vi "sort circles.vi"(1 "circles":T1(array[cluster])) -> (0 "Sorted circles":T1(array[cluster]))   [LabVIEW 2010]
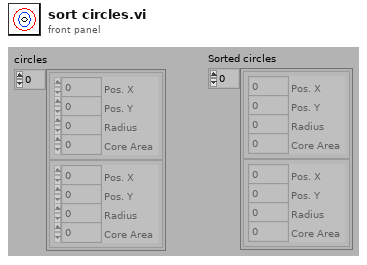
[diagram p1: front panel]
types:
  T1 = cluster{"Pos. X":i32, "Pos. Y":i32, "Radius":i32, "Core Area":i32}[]
  T2 = cluster{"Radius":i32, "Circles Data":cluster{"Pos. X":i32, "Pos. Y":i32, "Radius":i32, "Core Area":i32}}
  T3 = cluster{"Radius":i32, "Circles Data":cluster{"Pos. X":i32, "Pos. Y":i32, "Radius":i32, "Core Area":i32}}[]
  T4 = cluster{"Pos. X":i32, "Pos. Y":i32, "Radius":i32, "Core Area":i32}
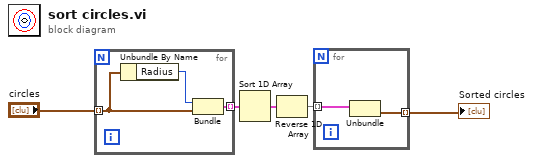
[diagram p0: block diagram]
diagram:
  n1 = for {
    tunnel: "circles" -> [w8] mode=indexing
    tunnel: [w7] -> w5 mode=indexing
    n2 = Unbundle By Name(w8) -> ("Radius"=w6:i32)
    n3 = Bundle("Radius"=w6, "Circles Data"=w8) -> (w7:T2)  [unwired: 1 in]
  }
  n4 = Sort 1D Array(array=w5) -> (sorted array=w4:T3)
  n5 = Reverse 1D Array(array=w4) -> (reversed array=w3:T3)
  n6 = for {
    tunnel: w3 -> [w10] mode=indexing
    tunnel: [w9] -> w1 mode=indexing
    n7 = Unbundle(w10) -> ("Circles Data"=w9:T4)  [unwired: 1 out]
  }
  "Sorted circles" <- w1
